vi "Test My Cloneable Module API.vi"() -> ()   [LabVIEW 2017]
doc: "My Module API Tester.\n_____\nBased on Delacor QMH Project Template 3.1.0.34."
uses:
  My Cloneable Module.lvlib
panel:
  in  "Run as Singleton?":bool
  in  "Show Block Diagram":bool
  in  "Refresh Modules":bool
  in  "X":dbl=1.0
  out "Reply Payload":dbl
  out "Reply Received?":bool
  out "Active Modules":string[](array[string])
  in  "Stop Module":bool
  in  "Select Module":i32(ring)=-1 caption="Select Module\nTo send Request to" items=["All"=-1]
  in  "Run New Module":bool
  out "Do Something Count":i32
  in  "Test Do Something Else and Wait for Reply":bool
  in  "Hide Module Panel":bool
  in  "Show Module Panel":bool
  in  "Test Do Something Else":bool
  in  "Test Do Something":bool
  out "Status":string
  # "This VI tests the API for the Module."
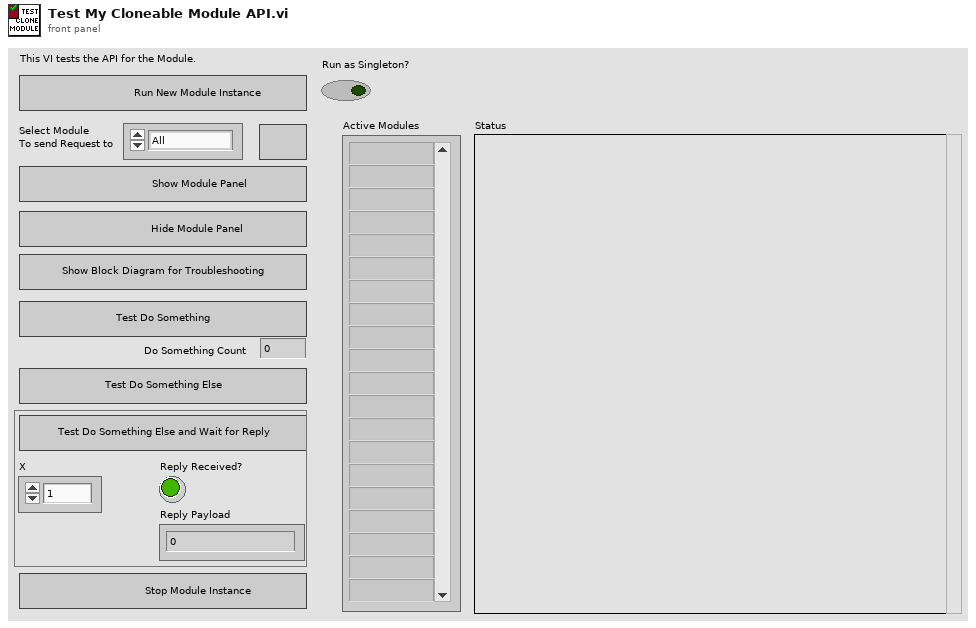
[diagram p1: front panel]
types:
  T1 = typedef "My Cloneable Module.lvlib/Broadcast Events--cluster.ctl" = cluster{"Module Did Init":refnum<user-event>, "Status Updated":refnum<user-event>, "Error Reported":refnum<user-event>, "Did Something":refnum<user-event>, "Module Did Stop":refnum<user-event>, "Update Module Execution Status":refnum<user-event>}
  T2 = typedef "My Cloneable Module.lvlib/Do Something Else and Wait (Reply Payload)--cluster.ctl" = cluster{"Value":dbl, "error":errorcluster}
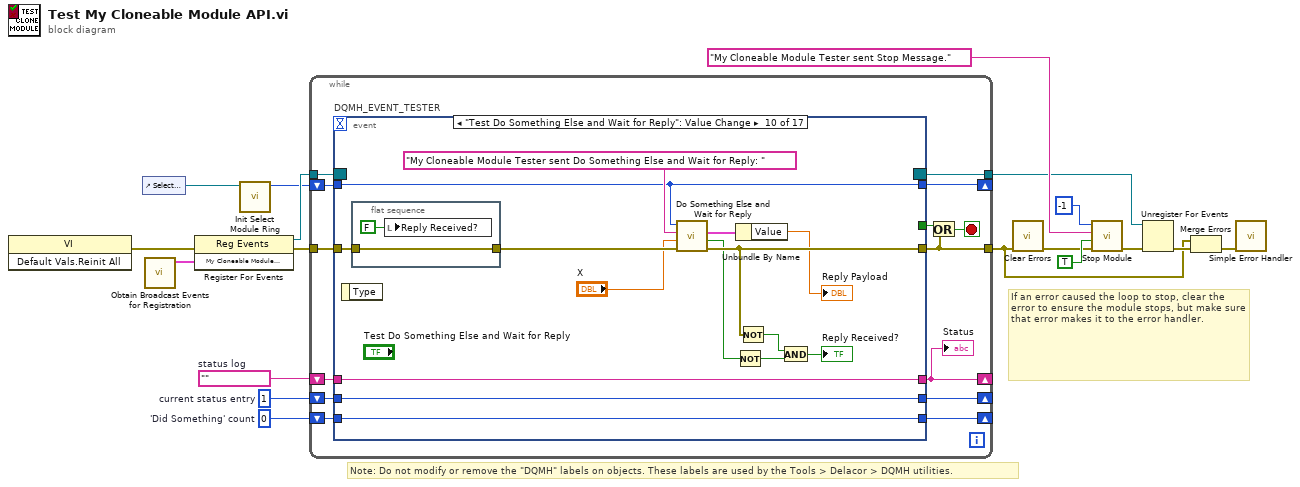
[diagram p0: block diagram]
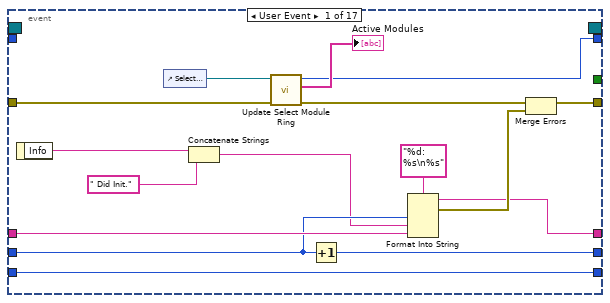
[diagram p2: hidden frame]
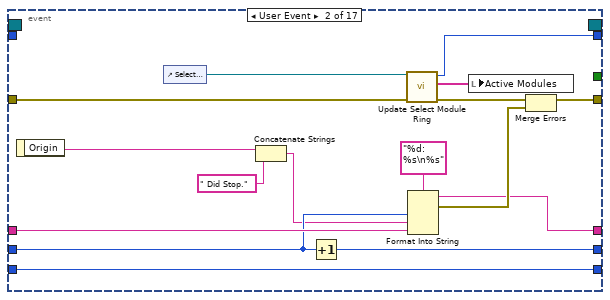
[diagram p3: hidden frame]
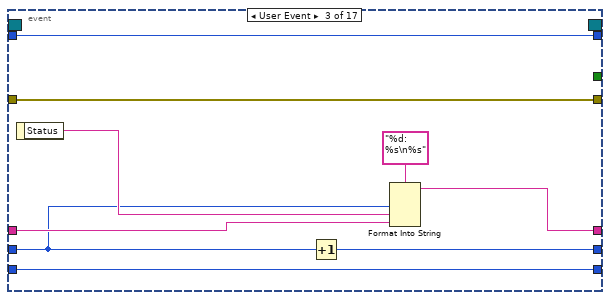
[diagram p4: hidden frame]
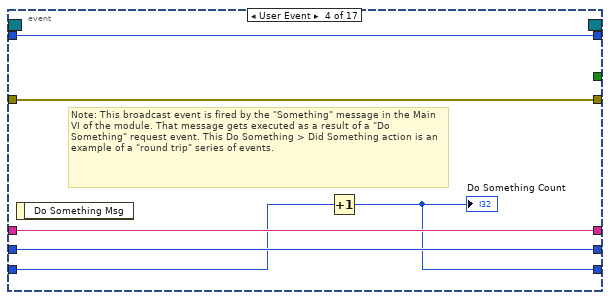
[diagram p5: hidden frame]
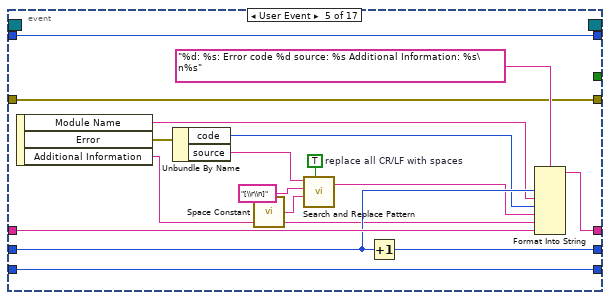
[diagram p6: hidden frame]
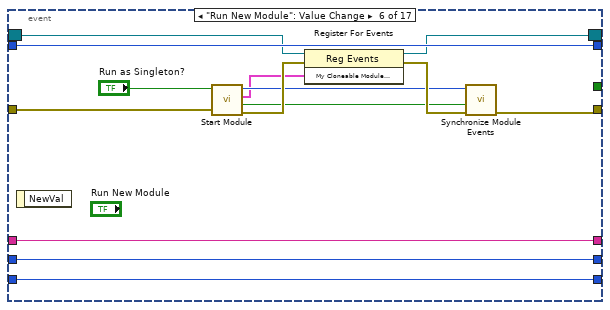
[diagram p7: hidden frame]
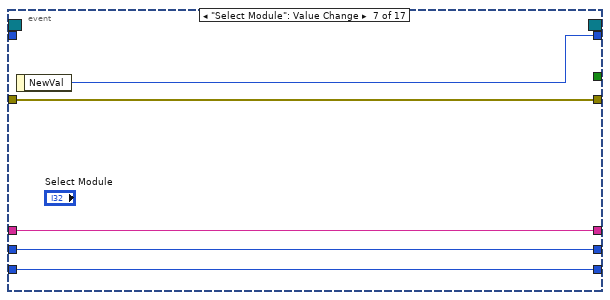
[diagram p8: hidden frame]
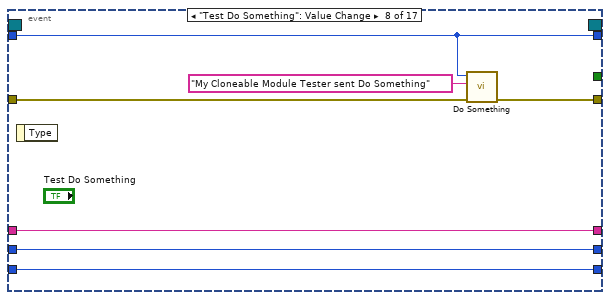
[diagram p9: hidden frame]
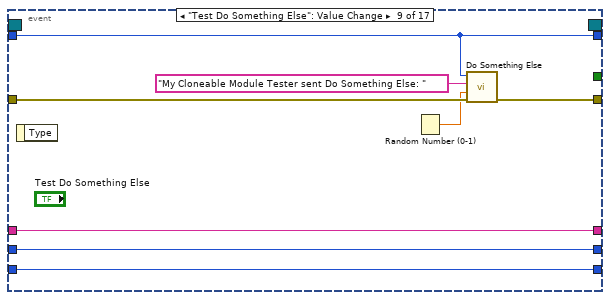
[diagram p10: hidden frame]
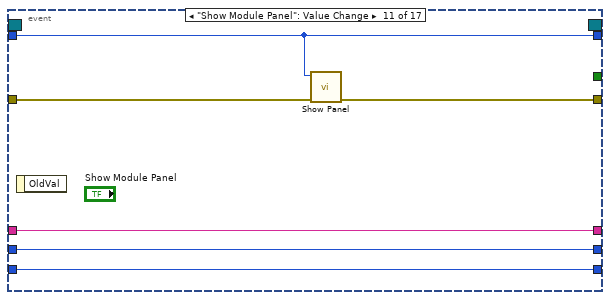
[diagram p11: hidden frame]
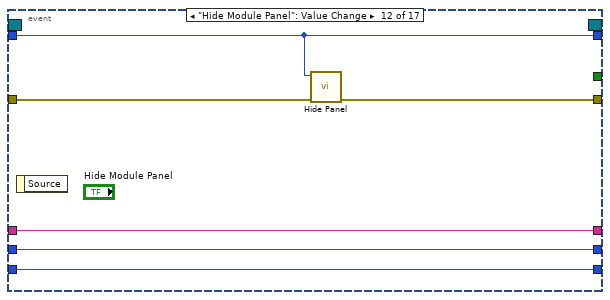
[diagram p12: hidden frame]
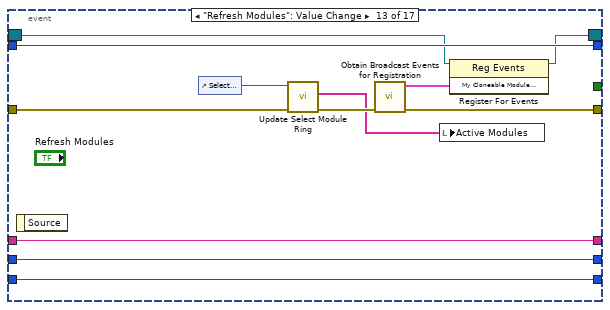
[diagram p13: hidden frame]
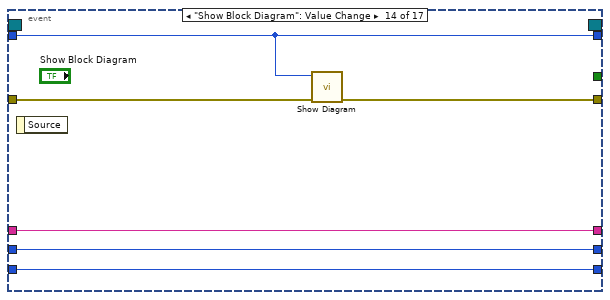
[diagram p14: hidden frame]
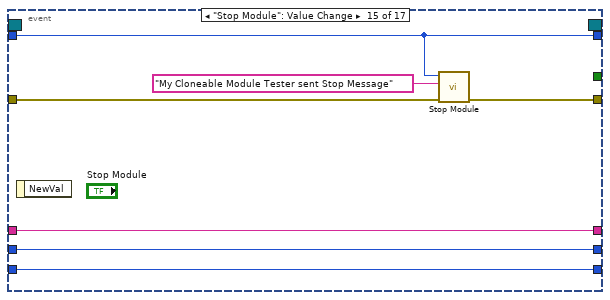
[diagram p15: hidden frame]
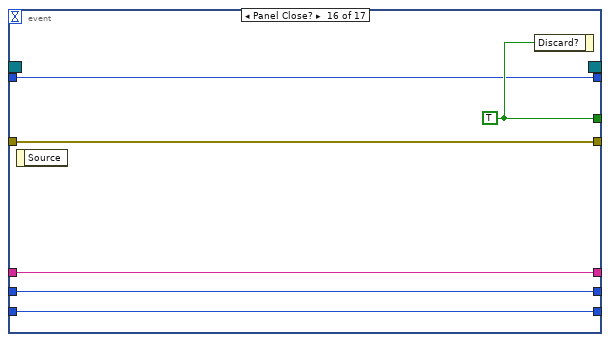
[diagram p16: hidden frame]
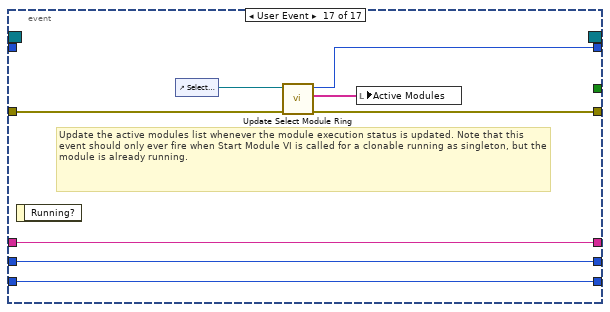
[diagram p17: hidden frame]
diagram:
  w13 = 0  # 'Did Something' count
  w14 = 1  # current status entry
  w15 = ""  # status log
  # "If an error caused the loop to stop, clear the error to ensure the module stops, but make sure that error makes it to the error handler."
  # "Note: Do not modify or remove the \"DQMH\" labels on objects. These labels are used by the Tools > Delacor > DQMH utilities."
  n1 = invoke class="VI" method="Default Vals.Reinit All"() -> (error out=w6:errorcluster)  [unwired: 3 in, 2 out]
  n2 = control-ref of="Select Module"() -> (w11:refnum<vi>)
  n3 = call "Obtain Broadcast Events for Registration.vi"() -> ("My Cloneable Module Broadcast Events"=w10:T1)  [unwired: 10 in, 1 out]
  n4 = register-events(error in=w6, w10) -> (reference out=w18:refnum<event-registration>, error out=w9:errorcluster)  [unwired: 1 in]
  n5 = call "Init Select Module Ring.vi"("Select Module Ring Ref"=w11) -> ("Value for All Modules"=w12:i32)  [unwired: 8 in, 2 out]
  n6 = while {
    tunnel: w18 -> [w32]
    tunnel: [w19] -> w1
    tunnel: w9 -> [w30]
    shift-right: [w26] -> _
    shift-left: w15 -> [w28]
    shift-right: [w27] -> _
    shift-left: w14 -> [w29]
    shift-right: [w24] -> _
    shift-left: w13 -> [w25]
    shift-right: [w21] -> _
    shift-left: w12 -> [w22]
    tunnel: [w20] -> w5
    stop <- w23 stop-if-true
    n7 = event "DQMH_EVENT_TESTER" shown="[9] \"Test Do Something Else and Wait for Reply\": Value Change" {
      selector: w32 -> [_ _ _ _ _ w103 _ _ _ _ _ _ w165 _ _ _ _]
      dyn-events: [_ _ _ _ _ w102 _ _ _ _ _ _ w164 _ _ _ _] -> w20
      timeout: _ -> [_ _ _ _ _ _ _ _ _ _ _ _ _ _ _ _ _]
      tunnel: [_ _ _ _ _ _ _ _ _ _ _ _ _ _ _ w190 _] -> w31
      tunnel: [w36 w55 w73 w79 w85 w101 w115 w121 w129 w145 w152 w158 w161 w173 w179 w189 w193] -> w19
      tunnel: w30 -> [w38 w57 w73 w79 w85 w104 w115 w122 w130 w136 w153 w159 w166 w177 w180 w189 w194]
      tunnel: w29 -> [w45 w61 w65 w77 w91 w107 w113 w118 w125 w142 w150 w156 w170 w175 w183 w187 w197]
      tunnel: w28 -> [w46 w62 w69 w78 w93 w108 w114 w119 w126 w143 w151 w157 w171 w176 w184 w188 w198]
      tunnel: [w43 w59 w70 w78 w88 w108 w114 w119 w126 w143 w151 w157 w171 w176 w184 w188 w198] -> w26
      tunnel: [w44 w60 w72 w77 w94 w107 w113 w118 w125 w142 w150 w156 w170 w175 w183 w187 w197] -> w27
      tunnel: w25 -> [w39 w58 w68 w76 w96 w106 w112 w117 w124 w141 w149 w155 w169 w174 w182 w186 w196]
      tunnel: [w39 w58 w68 w75 w96 w106 w112 w117 w124 w141 w149 w155 w169 w174 w182 w186 w196] -> w24
      tunnel: w22 -> [_ _ w66 w74 w95 w105 _ w116 w123 w140 w148 w154 w168 w172 w181 w185 _]
      tunnel: [w33 w52 w66 w74 w95 w105 w111 w116 w123 w140 w148 w154 w168 w172 w181 w185 w192] -> w21
      event User Event {
        n8 = event-data() -> ("Info"=w42:string)  [unwired: 1 in]
        n9 = control-ref of="Select Module"() -> (w35:refnum<vi>)
        n10 = Concatenate Strings(w42, " Did Init.") -> (w41:string)
        n11 = call "Update Select Module Ring.vi"("error in (no error)"=w38, "Select Module Ring Ref"=w35) -> ("error out"=w37:errorcluster, "Active Modules (Array)"=→"Active Modules":string[], "New Module Ring Value"=w33:i32)  [unwired: 7 in]
        n12 = Increment(x=w45) -> (x+1=w44:i32)
        n13 = Format Into String(format string="%d: %s\n%s", w45, w41, w46) -> (resulting string=w43:string, error out=w48:errorcluster)  [unwired: 2 in]
        n14 = Merge Errors(w37, w48) -> (w36:errorcluster)
      }
      event User Event {
        n15 = event-data() -> ("Origin"=w50:string)  [unwired: 1 in]
        n16 = control-ref of="Select Module"() -> (w54:refnum<vi>)
        n17 = Concatenate Strings(w50, " Did Stop.") -> (w49:string)
        n18 = Increment(x=w61) -> (x+1=w60:i32)
        n19 = call "Update Select Module Ring.vi"("error in (no error)"=w57, "Select Module Ring Ref"=w54) -> ("error out"=w56:errorcluster, "Active Modules (Array)"=w53:string[], "New Module Ring Value"=w52:i32)  [unwired: 7 in]
        n20 = Format Into String(format string="%d: %s\n%s", w61, w49, w62) -> (resulting string=w59:string, error out=w64:errorcluster)  [unwired: 2 in]
        n21 = local write "Active Modules"(w53) -> ()
        n22 = Merge Errors(w56, w64) -> (w55:errorcluster)
      }
      event User Event {
        n23 = event-data() -> ("Status"=w67:string)  [unwired: 1 in]
        n24 = Increment(x=w65) -> (x+1=w72:i32)
        n25 = Format Into String(format string="%d: %s\n%s", w65, w67, w69) -> (resulting string=w70:string)  [unwired: 2 in, 1 out]
      }
      event User Event {
        # "Note: This broadcast event is fired by the \"Something\" message in the Main VI of the module. That message gets executed as a result of a \"Do Something\" request event. This Do Something > Did Something action is an example of a \"round trip\" series of events."
        n26 = event-data() -> ()  [unwired: 1 in, 1 out]
        n27 = Increment(x=w76) -> (x+1=w75:i32)
        "Do Something Count" <- w75
      }
      event User Event {
        w89 = TRUE  # replace all CR/LF with spaces
        n28 = event-data() -> ("Module Name"=w83:string, "Error"=w82:errorcluster, "Additional Information"=w80:string)  [unwired: 1 in]
        n29 = Unbundle By Name(w82) -> ("code"=w84:i32, "source"=w86:string)
        n30 = call <vilib>:"Space Constant.vi"() -> ("String"=w90:string)
        n31 = call <vilib>:"Search and Replace Pattern.vi"("string"=w86, "regular expression (\"\")"="[\\r\\n]" ("regular expression (\"\")"), "replace string (\"\")"=w90, "replace all? (F)"=w89) -> ("result string"=w87:string)  [unwired: 1 in, 1 out]
        n32 = Increment(x=w91) -> (x+1=w94:i32)
        n33 = Format Into String(format string="%d: %s: Error code %d source: %s Additional Information: %s\n%s", w91, w83, w84, w87, w80, w93) -> (resulting string=w88:string)  [unwired: 2 in, 1 out]
      }
      event "Run New Module": Value Change {
        n34 = event-data() -> ()  [unwired: 1 in, 1 out]
        n35 = call "Start Module.vi"("error in (no error)"=w104, "Run as Singleton? (F)"="Run as Singleton?") -> ("error out"=w109:errorcluster, "Wait for Event Sync?"=w99:bool, "My Cloneable Module Broadcast Events"=w98:T1, "Module ID"=w100:i32)  [unwired: 6 in]
        n36 = register-events(reference=w103, error in=w109, w98) -> (reference out=w102:refnum<event-registration>, error out=w110:errorcluster)
        n37 = call "Synchronize Module Events.vi"("error in (no error)"=w110, "Wait for Event Sync?"=w99, "Module ID"=w100) -> ("error out"=w101:errorcluster)  [unwired: 7 in, 1 out]
      }
      event "Select Module": Value Change {
        n38 = event-data() -> ("NewVal"=w111:i32)  [unwired: 1 in]
      }
      event "Test Do Something": Value Change {
        n39 = event-data() -> ()  [unwired: 1 in, 1 out]
        n40 = call "Do Something.vi"("error in (no error)"=w122, "Do Something Message"="My Cloneable Module Tester sent Do Something", "Module ID"=w116) -> ("error out"=w121:errorcluster)  [unwired: 8 in]
      }
      event "Test Do Something Else": Value Change {
        n41 = event-data() -> ()  [unwired: 1 in, 1 out]
        n42 = Random Number (0-1)() -> (number: 0 to 1=w127:dbl)
        n43 = call "Do Something Else.vi"("error in (no error)"=w130, "X"=w127, "Do Something else Message"="My Cloneable Module Tester sent Do Something Else: " ("Do Something Message"), "Module ID"=w123) -> ("error out"=w129:errorcluster)  [unwired: 7 in]
      }
      event "Test Do Something Else and Wait for Reply": Value Change {
        n44 = event-data() -> ()  [unwired: 1 in, 1 out]
        n45 = flat-sequence {
          tunnel: w136 -> [w147]
          tunnel: [w147] -> w135
          frame #0 {
            n46 = local write "Reply Received?"(FALSE ("Reply Received?")) -> ()
          }
        }
        n47 = call "Do Something Else and Wait for Reply.vi"("error in (no error)"=w135, "X"="X", "Do Something Else Message"="My Cloneable Module Tester sent Do Something Else and Wait for Reply: " ("Do Something Message"), "Module ID"=w140) -> ("error out"=w145:errorcluster, "timed out?"=w137:bool, "Reply Payload"=w139:T2)  [unwired: 5 in]
        n48 = Not(x=w137) -> (.not. x?=w133:bool)
        n49 = Unbundle By Name(w139) -> ("Value"=→"Reply Payload":dbl)
        n50 = Not(x=w145) -> (.not. x?=w131:bool)
        n51 = And(x=w131, y=w133) -> (x .and. y?=→"Reply Received?":bool)
      }
      event "Show Module Panel": Value Change {
        n52 = event-data() -> ()  [unwired: 1 in, 1 out]
        n53 = call "Show Panel.vi"("error in (no error)"=w153, "Module ID"=w148) -> ("error out"=w152:errorcluster)  [unwired: 9 in]
      }
      event "Hide Module Panel": Value Change {
        n54 = event-data() -> ()  [unwired: 1 in, 1 out]
        n55 = call "Hide Panel.vi"("error in (no error)"=w159, "Module ID"=w154) -> ("error out"=w158:errorcluster)  [unwired: 9 in]
      }
      event "Refresh Modules": Value Change {
        n56 = event-data() -> ()  [unwired: 1 in, 1 out]
        n57 = control-ref of="Select Module"() -> (w167:refnum<vi>)
        n58 = call "Update Select Module Ring.vi"("error in (no error)"=w166, "Select Module Ring Ref"=w167) -> ("error out"=w162:errorcluster, "Active Modules (Array)"=w160:string[])  [unwired: 7 in, 1 out]
        n59 = call "Obtain Broadcast Events for Registration.vi"("error in (no error)"=w162) -> ("error out"=w161:errorcluster, "My Cloneable Module Broadcast Events"=w163:T1)  [unwired: 9 in]
        n60 = local write "Active Modules"(w160) -> ()
        n61 = register-events(reference=w165, w163) -> (reference out=w164:refnum<event-registration>)  [unwired: 1 in, 1 out]
      }
      event "Show Block Diagram": Value Change {
        n62 = event-data() -> ()  [unwired: 1 in, 1 out]
        n63 = call "Show Diagram.vi"("error in (no error)"=w177, "Module ID"=w172) -> ("error out"=w173:errorcluster)  [unwired: 9 in]
      }
      event "Stop Module": Value Change {
        n64 = event-data() -> ()  [unwired: 1 in, 1 out]
        n65 = call "Stop Module.vi"("error in (no error)"=w180, "Origin"="My Cloneable Module Tester sent Stop Message", "Module ID"=w181) -> ("error out"=w179:errorcluster)  [unwired: 8 in]
      }
      event Panel Close? {
        w190 = TRUE ("Discard?")
        n66 = event-data() -> ()  [unwired: 1 in, 1 out]
        n67 = event-data("Discard?"=w190) -> ()  [unwired: 1 in, 1 out]
      }
      event User Event {
        # "Update the active modules list whenever the module execution status is updated. Note that this event should only ever fire when Start Module VI is called for a clonable running as singleton, but the module is already running."
        n68 = event-data() -> ()  [unwired: 1 in, 1 out]
        n69 = control-ref of="Select Module"() -> (w195:refnum<vi>)
        n70 = call "Update Select Module Ring.vi"("error in (no error)"=w194, "Select Module Ring Ref"=w195) -> ("error out"=w193:errorcluster, "Active Modules (Array)"=w191:string[], "New Module Ring Value"=w192:i32)  [unwired: 7 in]
        n71 = local write "Active Modules"(w191) -> ()
      }
    }
    "Status" <- w26
    n72 = Or(x=w31, y=w19) -> (x .or. y?=w23:bool)
  }
  n73 = call <vilib>:"Clear Errors.vi"("error in (no error)"=w1) -> ("error out"=w3:errorcluster)  [unwired: 5 in, 1 out]
  n74 = call "Stop Module.vi"("error in (no error)"=w3, "Wait for Module to stop? (F)"=TRUE ("Wait for Module to stop?"), "Origin"="My Cloneable Module Tester sent Stop Message.", "Module ID"=-1 ("Stop all")) -> ("error out"=w16:errorcluster)  [unwired: 7 in]
  n75 = Unregister For Events(event registration refnum=w5, error in=w16) -> (error out=w17:errorcluster)
  n76 = Merge Errors(w1, w17) -> (w2:errorcluster)
  n77 = call <vilib>:"Simple Error Handler.vi"("error in (no error)"=w2) -> ()  [unwired: 4 in, 5 out]
